vi "Run boolean function for autonmous.vi"(11 "Boolean Function":string) -> (3 "yes/no":bool)   [LabVIEW 2013]
uses:
  Robot Global Var.vi
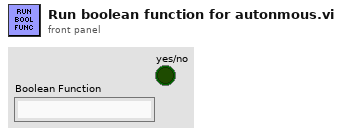
[diagram p1: front panel]
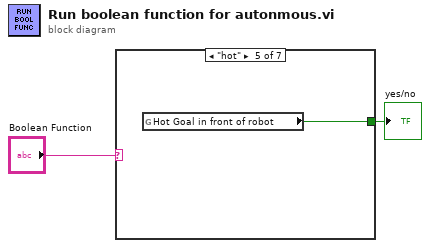
[diagram p0: block diagram]
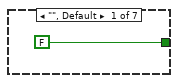
[diagram p2: hidden frame]
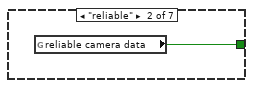
[diagram p3: hidden frame]
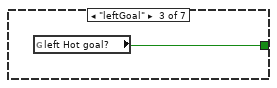
[diagram p4: hidden frame]
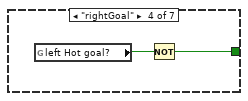
[diagram p5: hidden frame]
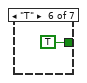
[diagram p6: hidden frame]
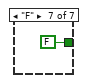
[diagram p7: hidden frame]
diagram:
  n1 = case shown="\"hot\"" "Boolean Function" {
    tunnel: [FALSE ("reliable camera data") w4 w5 w6 w8 TRUE ("left Hot goal?") FALSE ("left Hot goal?")] -> w1
    frame "", Default {
    }
    frame "reliable" {
      n2 = global read "Robot Global Var.vi" "reliable camera data"() -> (w4:bool)
    }
    frame "leftGoal" {
      n3 = global read "Robot Global Var.vi" "left Hot goal?"() -> (w5:bool)
    }
    frame "rightGoal" {
      n4 = global read "Robot Global Var.vi" "left Hot goal?"() -> (w7:bool)
      n5 = Not(x=w7) -> (.not. x?=w6:bool)
    }
    frame "hot" {
      n6 = global read "Robot Global Var.vi" "Hot Goal in front of robot"() -> (w8:bool)
    }
    frame "T" {
    }
    frame "F" {
    }
  }
  "yes/no" <- w1
